vi "Server Network Settings.vi"(8 "error in (no error)":errorcluster, 11 "Configuration in":refnum<class "Configuration.lvclass">) -> (0 "error out":errorcluster, 3 "Configuration out":refnum<class "Configuration.lvclass">)   [LabVIEW 2026, in "Server Controller.lvlib" / "Server Config.lvclass"]
uses:
  Server Config.lvclass
  configuration/Configuration.lvclass
  C:/Users/E2013170/Documents/GitHub/Measurement-Utility-Reference/source/configuration/Configuration.lvclass
  Server Config.lvclass/Server Config.ctl
panel:
  in  "Listener Port":u16
  in  "Context Name":string
  # "This only needs to be changed in the event that another server is\nrunning on the same machine, as they will need to have unique\ncontexts. Current connections will continue to use previous context.\nTo switch all clients to the new context, toggle the server off briefly\nto force clients to reconnect."
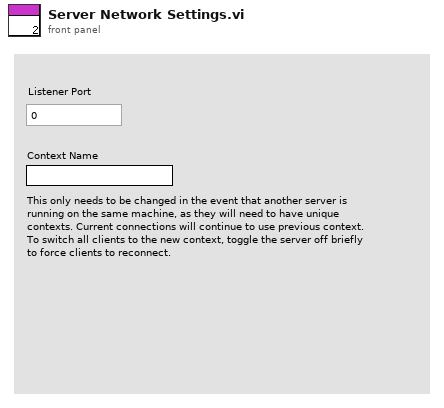
[diagram p1: front panel]
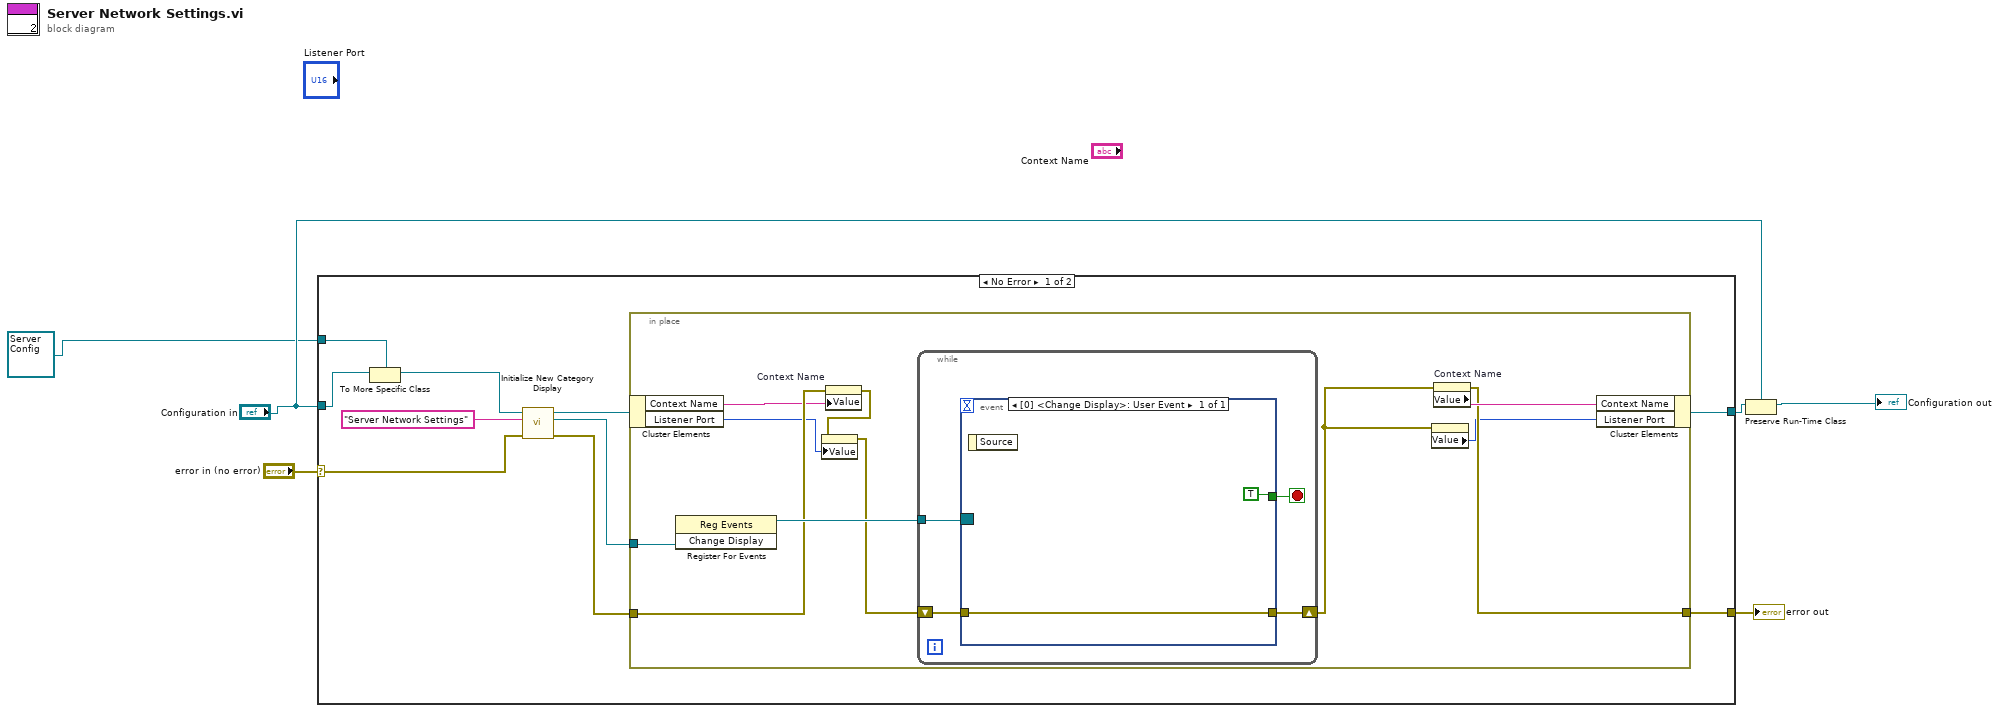
[diagram p0: block diagram]
diagram:
  n1 = case shown="No Error" "error in (no error)" {
    selector: "error in (no error)" -> [w12 w35]
    tunnel: [w11 w34] -> w3
    tunnel: [w14 w35] -> w6
    tunnel: "Configuration in" -> [w10 w34]
    tunnel: refnum<class "Server Config.lvclass"> refnum ("Server Controller.lvlib:Server Config.lvclass") -> [w8 _]
    frame No Error {
      n2 = To More Specific Class(target class=w8, reference=w10) -> (specific class reference=w9:refnum<class "Server Config.lvclass">)  [unwired: 1 in, 1 out]
      n3 = call "Initialize New Category Display.vi"("error in (no error)"=w12, "Name to Display"="Server Network Settings", "Configuration in"=w9) -> ("error out"=w15:errorcluster, "Change Display"=w16:refnum<user-event>, "Configuration Out"=w7:refnum<class "Server Config.lvclass">)  [unwired: 6 in]
      n4 = in-place {
        in-place-border: w16 -> [w27]
        in-place-border: w15 -> [w25]
        in-place-border: [w23] -> w14
        n5 = in-place-cluster #1(w7) -> ("Context Name"=w18:string, "Listener Port"=w17:u16)
        n6 = register-events(w27) -> (reference out=w26:refnum<event-registration>)  [unwired: 2 in, 1 out]
        n7 = property on="Context Name" class="Str"(error in=w25, "Value"=w18) -> (error out=w22:errorcluster)  [unwired: 1 in, 1 out]
        n8 = property on="Listener Port" class="DigNum (strict)"(error in=w22, "Value"=w17) -> (error out=w21:errorcluster)  [unwired: 1 in, 1 out]
        n9 = while {
          tunnel: w26 -> [w30]
          shift-right: [w29] -> w19
          shift-left: w21 -> [w28]
          stop <- w31 stop-if-true
          n10 = event shown="[0] <Change Display>: User Event" {
            selector: w30 -> [_]
            dyn-events: _ -> [_]
            timeout: _ -> [_]
            tunnel: [TRUE] -> w31
            tunnel: [w32] -> w29
            tunnel: w28 -> [w32]
            event User Event {
              n11 = event-data() -> ()  [unwired: 1 in, 1 out]
            }
          }
        }
        n12 = property on="Listener Port" class="DigNum (strict)"(error in=w19) -> ("Value"=w20:u16)  [unwired: 1 in, 2 out]
        n13 = property on="Context Name" class="Str"(error in=w19) -> (error out=w23:errorcluster, "Value"=w24:string)  [unwired: 1 in, 1 out]
        n14 = in-place-cluster #1("Context Name"=w24, "Listener Port"=w20) -> (w11:refnum<class "Server Config.lvclass">)
      }
    }
    frame Error {
    }
  }
  "error out" <- w6
  n15 = Preserve Run-Time Class(object in=w3, 2:"Configuration in") -> (object out=→"Configuration out":refnum<class "Configuration.lvclass">)  [unwired: 1 in, 1 out]
